vi "to string.vi"(8 "error in":errorcluster, 11 "SystemLin Tag Module configuration in":refnum<class "SystemLink File configuration.lvclass">) -> (0 "error out":errorcluster, 1 "data":string, 2 "version":string, 3 "SystemLin Tag Module configuration out":refnum<class "SystemLink File configuration.lvclass">)   [LabVIEW 2015, in "SystemLink File configuration.lvclass"]
doc: "Provides an interface for saving a module configuration to a file or other serialized data source. It is recommended that all children of this class store data in two sets--data required for its own initialization, and any data required for parent initialization--and that each implementation uses the <b>Call Parent Method</b> primitive to serialize parent information."
uses:
  SystemLink File configuration.lvclass
  SystemLink File configuration.lvclass/SystemLink File configuration.ctl
  current version.vi
  <vilib>/NI/Tag Bus Module Framework/module configuration/TBM module configuration.lvclass
  <vilib>/NI/Tag Bus Module Framework/channel/TBM channel.lvclass
  <vilib>/NI/Configuration Framework/serializable configuration/NISE_CEF_serializable configuration.lvclass
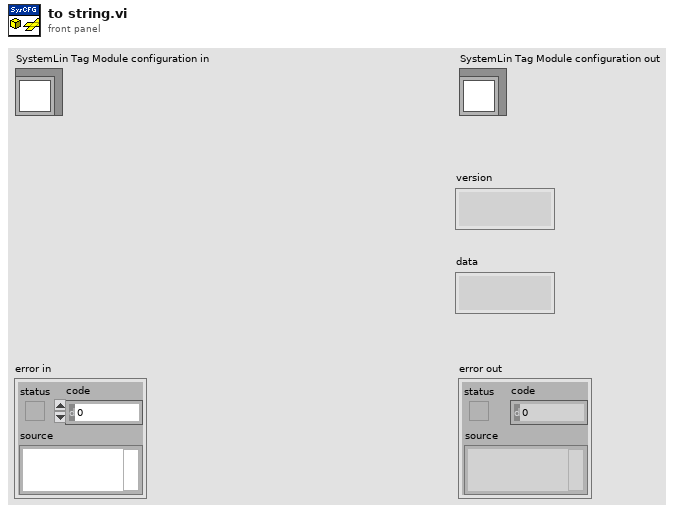
[diagram p1: front panel]
types:
  T1 = typedef "SystemLink File configuration.lvclass/Connection Configuration.ctl" = cluster{"Connection Type":T2, "AMQP":cluster{"Configuration ID":string}, "HTTP":cluster{"Verify Server?":bool, "Server URL":string, "CA Certificate File":string, "User Info":cluster{"Username":string, "Password":string}, "API Key":string}}
  T2 = typedef "SystemLink File configuration.lvclass/Connection Type.ctl" = enum16{"AMQP", "HTTP", "API Key (SystemLink Cloud)"}
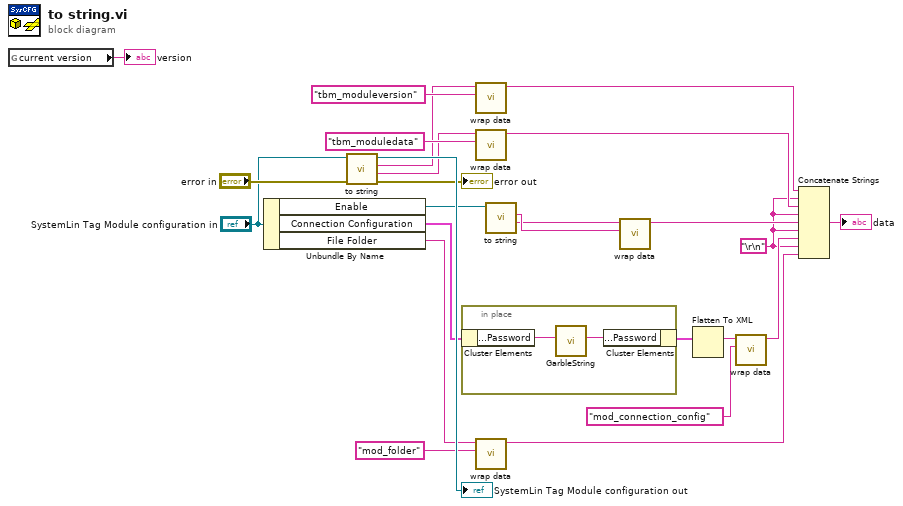
[diagram p0: block diagram]
diagram:
  w6 = "\r\n"
  n1 = global read "current version.vi" "current version"() -> (→"version":string)
  n2 = Unbundle By Name("SystemLin Tag Module configuration in") -> ("Enable"=w7:refnum<class "TBM channel.lvclass">, "Connection Configuration"=w8:T1, "File Folder"=w3:string)
  n3 = call-parent "to string.vi"("error in"="error in", "module configuration in"="SystemLin Tag Module configuration in") -> ("error out"=→"error out":errorcluster, "data"=w16:string, "version"=w17:string, "module configuration out"=→"SystemLin Tag Module configuration out":refnum<class "SystemLink File configuration.lvclass">)  [unwired: 6 in]
  n4 = in-place {
    n5 = in-place-cluster #1(w8) -> ("HTTP.User Info.Password"=w27:string)
    n6 = call "GarbleString.vi"("String In"=w27) -> ("String Out"=w26:string)  [unwired: 10 in]
    n7 = in-place-cluster #1("HTTP.User Info.Password"=w26) -> (w10:T1)
  }
  n8 = call <vilib>:"wrap data.vi"("identifier"="tbm_moduleversion" ("additional identifier"), "data to wrap"=w17) -> ("wrapped data"=w19:string)  [unwired: 9 in]
  n9 = call <vilib>:"wrap data.vi"("identifier"="tbm_moduledata" ("additional identifier"), "data to wrap"=w16) -> ("wrapped data"=w18:string)  [unwired: 9 in]
  n10 = call <vilib>:"wrap data.vi"("identifier"="mod_folder", "data to wrap"=w3) -> ("wrapped data"=w5:string)  [unwired: 9 in]
  n11 = call-dynamic "to string.vi"("channel in"=w7) -> ("channel data"=w1:string, "identifier"=w2:string)  [unwired: 7 in, 2 out]
  n12 = call <vilib>:"wrap data.vi"("identifier"=w2, "data to wrap"=w1) -> ("wrapped data"=w14:string)  [unwired: 9 in]
  n13 = Flatten To XML(anything=w10) -> (xml string=w13:string)
  n14 = call <vilib>:"wrap data.vi"("identifier"="mod_connection_config", "data to wrap"=w13) -> ("wrapped data"=w12:string)  [unwired: 9 in]
  n15 = Concatenate Strings(w19, w6, w18, w6, w14, w6, w12, w6, w5) -> (→"data":string)
